vi "Renishaw-XL80_GetLaserMeasurement.vi"(8 "error in (no error)":errorcluster, 11 "Renishaw-XL80_EMU in":refnum<class "Renishaw-XL80_EMU.lvclass">) -> (0 "error out":errorcluster, 1 "pStatus":i32(ring) items=["COUNT_OK"=0, "COUNT_ERROR"=1, "COUNT_TPIN_OCCURRED"=2, "COUNT_DATUMED"=4], 2 "GetLaserMeasurement":dbl, 3 "Renishaw-XL80_EMU out":refnum<class "Renishaw-XL80_EMU.lvclass">)   [LabVIEW 2024, in "Renishaw-XL80_EMU.lvclass"]
doc: "This method retrieves the latest laser reading. The units for this reading depend upon the measurement mode. For linear and straightness modes the reading is in m. For angular the reading is in radians.\n\nDefinition\nHRESULTGetLaserMeasurement( [out] COUNT_STATUS_CODES *pStatus, [out, retval] double *pVal);\nParameters\npStatus\nA variable that will be set to the COUNT_STATUS_CODES.\n\npVal\nA variable that will be set to the laser measurement (in m or in rad).\n\nComments\nThis method will return with an HRESULT of E_FAIL if the client has not previously connected to a DX10 by calling Connect. The method will also return E_FAIL if the DX10 is not responding.\n\nThe property will normally return an HRESULT of S_OK. However, it will return E_POINTER if the client supplies a null pointer for either pVal or pStatus.\n\nIf the DX10 is responding but the ML10 is not responding, then the last received reading will be retrieved.\n\nThe reading is affected by the MeasurementMode, OpticsFactor, Lambda, and MatCompFactor"
uses:
  Renishaw-XL80_EMU.lvclass
  <vilib>/numeric/Random Number (Range) U64.vi
  <vilib>/numeric/sub_Random U32.vi
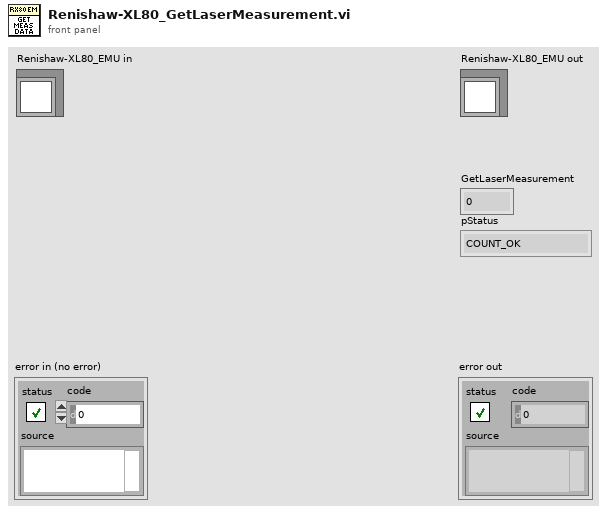
[diagram p1: front panel]
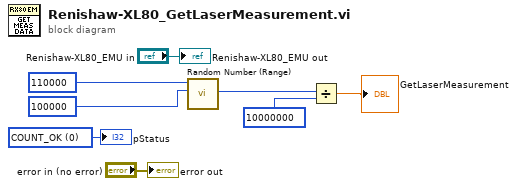
[diagram p0: block diagram]
diagram:
  w6 = 0 items=["COUNT_OK"=0, "COUNT_ERROR"=1, "COUNT_TPIN_OCCURRED"=2, "COUNT_DATUMED"=4] ("pStatus")
  n1 = call-poly <vilib>:"Random Number (Range).vi"("lower bound (0)"=u64 100000, "upper bound (100)"=u64 110000) -> ("number"=w3:u64)  [unwired: 9 in]
  n2 = Divide(x=w3, y=u64 10000000) -> (x/y=→"GetLaserMeasurement":dbl)
  "error out" <- "error in (no error)"
  "Renishaw-XL80_EMU out" <- "Renishaw-XL80_EMU in"
  "pStatus" <- w6
